vi "Paths Manager.vi"(8 "error in":errorcluster, 11 "Controller in":refnum<class "Controller.lvclass">) -> (0 "error out":errorcluster, 2 "Paths":T1, 3 "Controller out":refnum<class "Controller.lvclass">)   [LabVIEW 2022 SP3, in "Controller.lvlib" / "Controller.lvclass"]
uses:
  Controller.lvclass
  <vilib>/Utility/sysdir.llb/System Directory Type.ctl
  Controller.lvclass/Controller.ctl
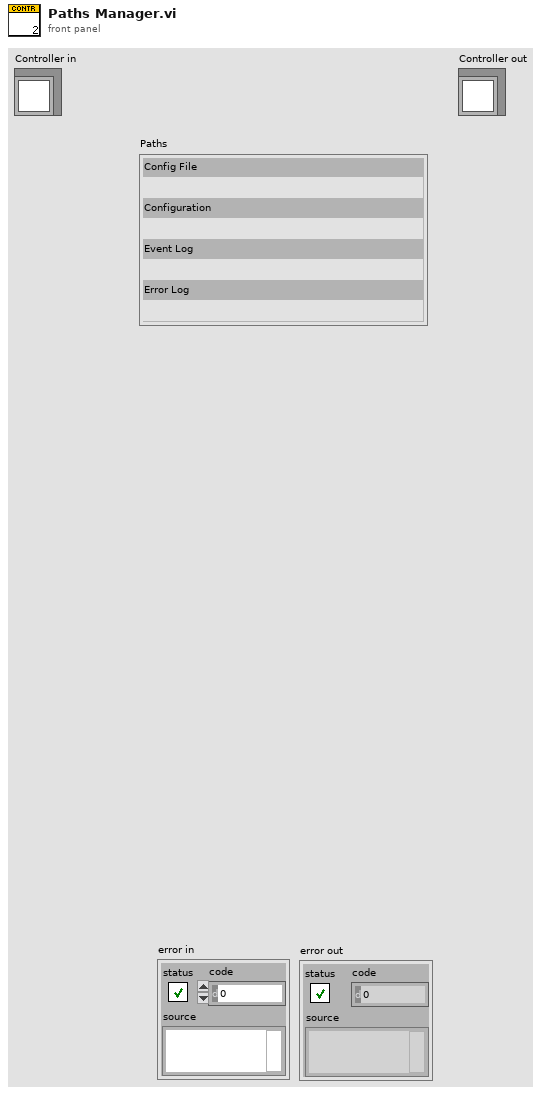
[diagram p1: front panel]
types:
  T1 = cluster{"Config File ":path, "Configuration":path, "Event Log":path, "Error Log":path}
  T2 = typedef "System Directory Type.ctl" = i32
  T3 = cluster{"File Array[0]":path, "File Array[1]":path, "File Array[2]":path, "File Array[3]":path, "File Array[4]":path, "File Array[5]":path, "File Array[6]":path, "File Array[7]":path, "File Array[8]":path}
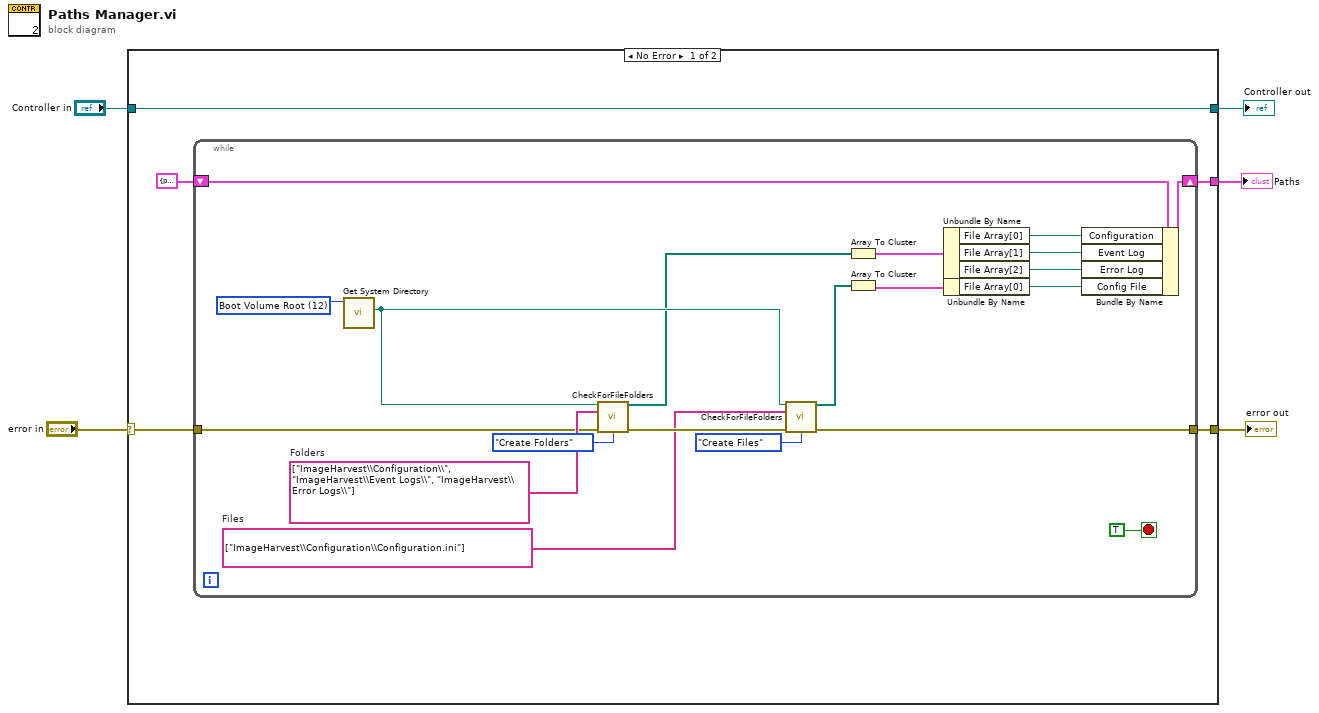
[diagram p0: block diagram]
diagram:
  n1 = case shown="No Error" "error in" {
    selector: "error in" -> [w9 w32]
    tunnel: [w8 w32] -> w4
    tunnel: [w6 w31] -> w2
    tunnel: "Controller in" -> [w6 w31]
    tunnel: [w10 _] -> w1
    frame No Error {
      n2 = while {
        shift-right: [w17] -> w10
        shift-left: T1 {"Config File "=path "", "Configuration"=path "", "Event Log"=path "", "Error Log"=path ""} ("Paths") -> [w20]
        tunnel: w9 -> [w26]
        tunnel: [w24] -> w8
        stop <- TRUE stop-if-true
        w29 = T2 12 items=["User Home"=0, "User Desktop"=1, "User Documents"=2, "User Application Data"=3, "User Preferences"=4, "User Temporary"=5, "Public Documents"=6, "Public Application Data"=7, "Public Preferences"=8, "Public Cache"=13, "System Core Libraries"=9, "System Installed Libraries"=10, "Application Files"=11, "Boot Volume Root"=12] ("system directory type")
        w22 = string[] ["ImageHarvest\\Configuration\\Configuration.ini"]  # Files
        w28 = string[] ["ImageHarvest\\Configuration\\", "ImageHarvest\\Event Logs\\", "ImageHarvest\\Error Logs\\"]  # Folders
        n3 = call <vilib>:"Get System Directory.vi"("system directory type"=w29) -> ("system directory"=w23:path)  [unwired: 10 in]
        n4 = call "CheckForFileFolders.vi"("Main Path"=w23, "Sub Path"=w28, "Error in (no error)"=w26, "Operation"=enum16{"Create Files", "Create Folders"}."Create Folders") -> ("File Array"=w19:path[], "Error out"=w25:errorcluster)  [unwired: 10 in]
        n5 = call "CheckForFileFolders.vi"("Main Path"=w23, "Sub Path"=w22, "Error in (no error)"=w25, "Operation"=enum16{"Create Files", "Create Folders"}."Create Files") -> ("File Array"=w16:path[], "Error out"=w24:errorcluster)  [unwired: 10 in]
        n6 = Array To Cluster(array=w19) -> (cluster=w18:T3)
        n7 = Array To Cluster(array=w16) -> (cluster=w15:T3)
        n8 = Unbundle By Name(w18) -> ("File Array[0]"=w13:path, "File Array[1]"=w12:path, "File Array[2]"=w11:path)
        n9 = Unbundle By Name(w15) -> ("File Array[0]"=w14:path)
        n10 = Bundle By Name(cluster=w20, "Configuration"=w13, "Event Log"=w12, "Error Log"=w11, "Config File"=w14) -> (w17:T1)
      }
    }
    frame Error {
    }
  }
  "error out" <- w4
  "Controller out" <- w2
  "Paths" <- w1
